vi "Store Configuration Parameters.vi"(8 "error in (no error)":errorcluster, 10 "refnum":T1, 11 "Motions Configuration in":refnum<class "Motions Configuration.lvclass">) -> (0 "error out":errorcluster, 2 "refnum out":T1, 3 "Motions Configuration out":refnum<class "Motions Configuration.lvclass">)   [LabVIEW 2016, in "Hardware.lvlib" / "Motions.lvlib" / "Motions Configuration.lvclass"]
uses:
  <userlib>/Common Components/Hardware/Abstract System/Motions/Motions Config/Motions Configuration.lvclass
  <vilib>/Utility/config.llb/Config Data RefNum.ctl
  <userlib>/Configuration Dialog Actor/Configuration.lvclass
  <userlib>/Common Components/Hardware/Motor/Motor Config/Motor Configuration.lvclass
  <vilib>/Utility/config.llb/NI_LVConfig.lvlib
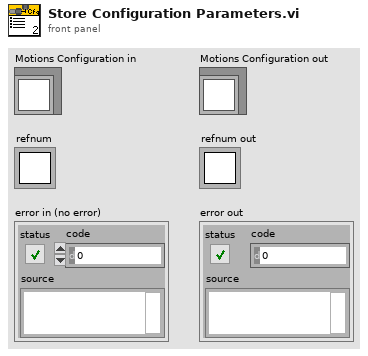
[diagram p1: front panel]
types:
  T1 = typedef "NI_LVConfig.lvlib/Config Data RefNum.ctl" = refnum<k1>
  T2 = typedef "Hardware.lvlib/Motions.lvlib/Motions.lvclass/TA Binding Data.ctl" = cluster{"Triggers":cluster{"Triggers for Array AND":cluster{"Index":u8, "State Name":string}[]}[], "Actions":cluster{"Action Name":string, "Action Data":string}[]}
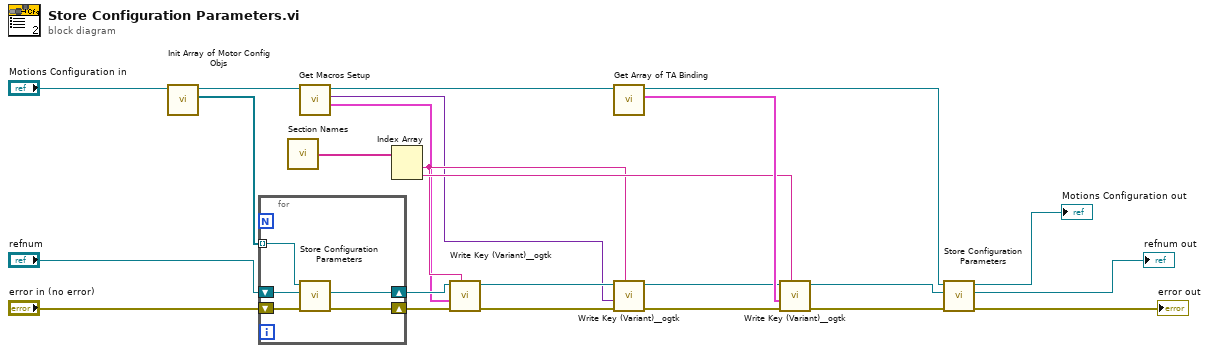
[diagram p0: block diagram]
diagram:
  n1 = call <userlib>:"Init Array of Motor Config Objs.vi"("Motions Configuration in"="Motions Configuration in") -> ("Array of Motor Config Objs"=w19:refnum<class "Motor Configuration.lvclass">[], "Motions Configuration out"=w20:refnum<class "Motions Configuration.lvclass">)  [unwired: 8 in, 1 out]
  n2 = for {
    tunnel: w19 -> [w29] mode=indexing
    shift-right: [w27] -> w12
    shift-left: "refnum" -> [w28]
    shift-right: [w25] -> w16
    shift-left: "error in (no error)" -> [w26]
    n3 = call-dynamic "Store Configuration Parameters.vi"("error in (no error)"=w26, "refnum"=w28, "Example Configuration Dialog in"=w29) -> ("error out"=w25:errorcluster, "refnum out"=w27:T1)  [unwired: 6 in, 1 out]
  }
  n4 = call <userlib>:"Section Names.vi"() -> ("Array of Section Names"=w10:string[])
  n5 = call <userlib>:"Get Macros Setup.vi"("Motions Configuration in"=w20) -> ("Macros List"=w2:cluster{"enabled?":bool, "macro name":string}[], "Macro LUT (Name->Macro)"=w1:variant, "Motions Configuration out"=w7:refnum<class "Motions Configuration.lvclass">)  [unwired: 7 in, 1 out]
  n6 = Index Array(array=w10) -> (element #1=w3:string, element #2=w8:string)  [unwired: 2 in]
  n7 = call <userlib>:"Write Key (Variant)__ogtk.vi"("section"=w3, "error in (no error)"=w16, "key-value"=w2, "refnum"=w12) -> ("error out"=w13:errorcluster, "refnum out"=w5:T1)  [unwired: 6 in]
  n8 = call <userlib>:"Get Array of TA Binding.vi"("Motions Configuration in"=w7) -> ("Array of TA Binding"=w9:T2[], "Motions Configuration out"=w11:refnum<class "Motions Configuration.lvclass">)  [unwired: 8 in, 1 out]
  n9 = call <userlib>:"Write Key (Variant)__ogtk.vi"("section"=w3, "error in (no error)"=w13, "key-value"=w1, "refnum"=w5) -> ("error out"=w6:errorcluster, "refnum out"=w4:T1)  [unwired: 6 in]
  n10 = call <userlib>:"Write Key (Variant)__ogtk.vi"("section"=w8, "error in (no error)"=w6, "key-value"=w9, "refnum"=w4) -> ("error out"=w15:errorcluster, "refnum out"=w14:T1)  [unwired: 6 in]
  n11 = call-parent "Store Configuration Parameters.vi"("error in (no error)"=w15, "refnum"=w14, "Configuration in"=w11) -> ("error out"=→"error out":errorcluster, "refnum out"=→"refnum out":T1, "Configuration out"=→"Motions Configuration out":refnum<class "Motions Configuration.lvclass">)  [unwired: 6 in]
